vi "Test Assert Array Distinct.vi"(8 "error in (no error)":errorcluster) -> (0 "error out":errorcluster)   [LabVIEW 2013]
uses:
  classes/Assert/Assert.lvclass
  classes/Test/Test.lvclass
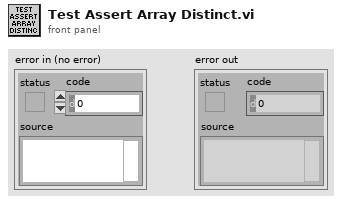
[diagram p1: front panel]
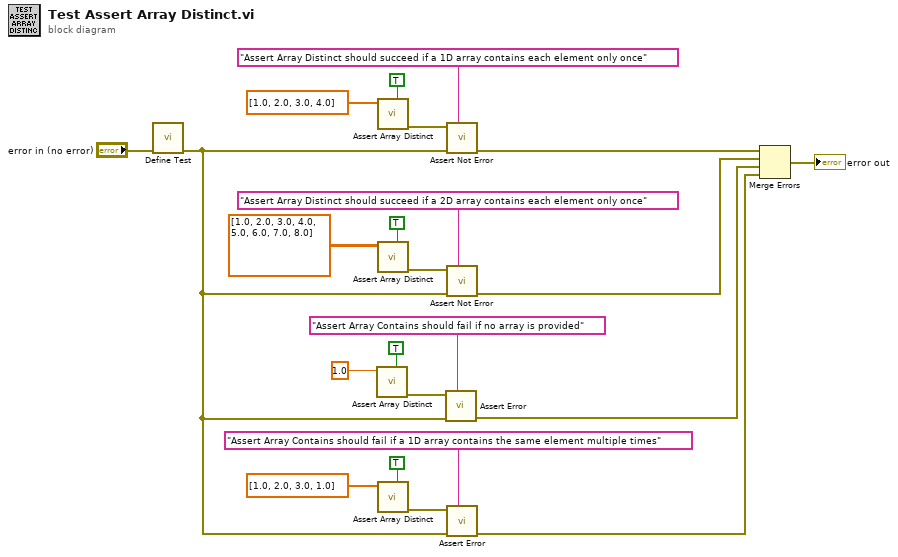
[diagram p0: block diagram]
diagram:
  n1 = call "Define Test.vi"("error in (no error)"="error in (no error)") -> ("error out"=w7:errorcluster)  [unwired: 9 in, 1 out]
  n2 = call "Assert Array Distinct.vi"("Assert Only? (F)"=TRUE, "Array"=1.0 ("element")) -> ("error out"=w11:errorcluster)  [unwired: 8 in, 1 out]
  n3 = call "Assert Array Distinct.vi"("Assert Only? (F)"=TRUE, "Array"=dbl[] [1.0, 2.0, 3.0, 4.0] ("initialized array")) -> ("error out"=w23:errorcluster)  [unwired: 8 in, 1 out]
  n4 = call "Assert Array Distinct.vi"("Assert Only? (F)"=TRUE, "Array"=dbl[][] [[1.0, 2.0, 3.0, 4.0], [5.0, 6.0, 7.0, 8.0]] ("initialized array")) -> ("error out"=w15:errorcluster)  [unwired: 8 in, 1 out]
  n5 = call "Assert Array Distinct.vi"("Assert Only? (F)"=TRUE, "Array"=dbl[] [1.0, 2.0, 3.0, 1.0] ("initialized array")) -> ("error out"=w1:errorcluster)  [unwired: 8 in, 1 out]
  n6 = call "Assert Error.vi"("Label"="Assert Array Contains should fail if no array is provided", "error in (no error)"=w7, "Error?"=w11) -> ("error out"=w9:errorcluster)  [unwired: 7 in, 1 out]
  n7 = call "Assert Not Error.vi"("Label"="Assert Array Distinct should succeed if a 1D array contains each element only once", "error in (no error)"=w7, "Not Error?"=w23) -> ("error out"=w19:errorcluster)  [unwired: 7 in, 1 out]
  n8 = call "Assert Not Error.vi"("Label"="Assert Array Distinct should succeed if a 2D array contains each element only once", "error in (no error)"=w7, "Not Error?"=w15) -> ("error out"=w14:errorcluster)  [unwired: 7 in, 1 out]
  n9 = call "Assert Error.vi"("Label"="Assert Array Contains should fail if a 1D array contains the same element multiple times", "error in (no error)"=w7, "Error?"=w1) -> ("error out"=w6:errorcluster)  [unwired: 7 in, 1 out]
  n10 = Merge Errors(w19, w14, w9, w6) -> (→"error out":errorcluster)
